vi "callback_send.vi"(8 "error in (no error)":errorcluster, 9 "flags":i32, 10 "buffer":u8[](array[numeric]), 11 "socket":u64) -> (0 "error out":errorcluster, 2 "bytes send":i64)   [LabVIEW 2017, in "support.lvlib"]
doc: "Called when libssh2 wants to send data on the connection.\n\n<B>socket</B> is the socket to write to.\n<B>buffer</B> is the data to send.\n<B>flags</B> are the flags that would have been used by a send() call.\n\nReturns the number of bytes sent."
uses:
  support.lvlib
  ws2_32.dll
  libc.so.6
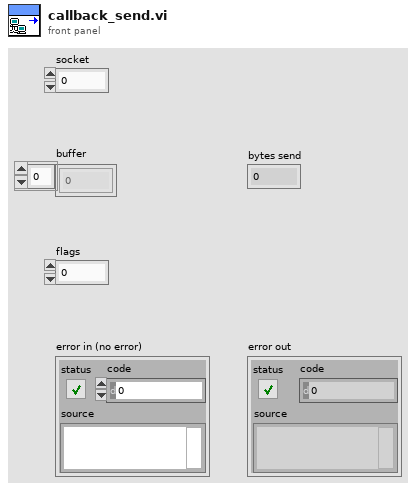
[diagram p1: front panel]
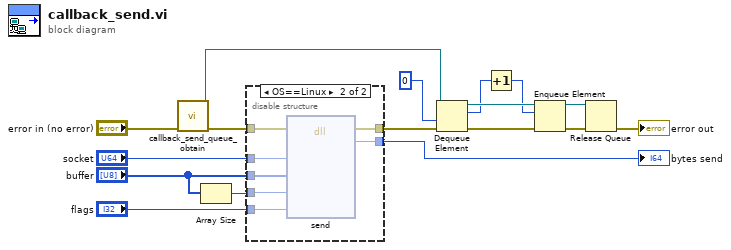
[diagram p0: block diagram]
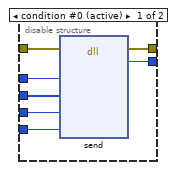
[diagram p2: hidden frame]
diagram:
  n1 = call "callback_send_queue_obtain.vi"("error in (no error)"="error in (no error)") -> ("error out"=w11:errorcluster, "queue out"=w9:refnum<queue>)  [unwired: 9 in]
  n2 = Array Size(array="buffer") -> (size(s)=w16:i32)
  n3 = disable-structure shown="OS==Linux" {
    disable-tunnel: "socket" -> [w24 w31]
    disable-tunnel: w16 -> [w23 w30]
    disable-tunnel: "buffer" -> [w22 w29]
    disable-tunnel: "flags" -> [w21 w28]
    disable-tunnel: [w20 w27] -> w13
    disable-tunnel: w11 -> [w19 w26]
    disable-tunnel: [w18 w25] -> w8
    frame condition #0 (active) {
      n4 = dll-call lib="ws2_32.dll" fn="send"(error in=w19, "s"=w24, "buf"=w22, "len"=w23, "flags"=w21) -> (error out=w20:errorcluster, "return type"=w18:i32)  [unwired: 6 in, 1 out]
    }
    frame condition #1 {
      n5 = dll-call lib="libc.so.6" fn="send"(error in=w26, "sockfd"=w31, "buf"=w29, "size"=w30, "flags"=w28) -> (error out=w27:errorcluster, "return type"=w25:i32)  [unwired: 6 in, 1 out]
    }
  }
  "bytes send" <- w8
  n6 = Dequeue Element(queue=w9, timeout in ms (-1)=0, error in (no error)=w13) -> (queue out=w3:refnum<queue>, element=w2:i64, error out=w10:errorcluster)  [unwired: 1 out]
  n7 = Increment(x=w2) -> (x+1=w1:i64)
  n8 = Enqueue Element(queue=w3, element=w1, error in (no error)=w10) -> (queue out=w4:refnum<queue>, error out=w5:errorcluster)  [unwired: 1 in, 1 out]
  n9 = Release Queue(queue=w4, error in (no error)=w5) -> (error out=→"error out":errorcluster)  [unwired: 1 in, 2 out]
